vi "Extract Capacity Rows.vi"(10 "Row":i32, 11 "all rows":string[][](array[string])) -> (3 "Capacity Data":T1)   [LabVIEW 2012]
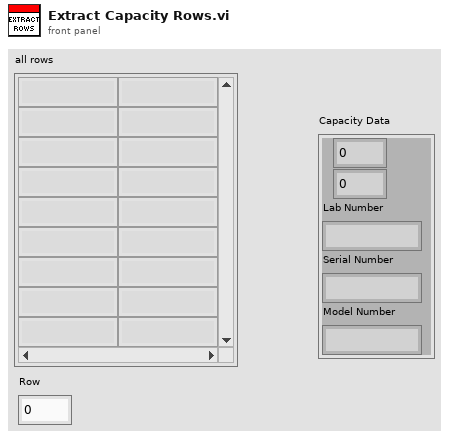
[diagram p1: front panel]
types:
  T1 = cluster{"Measured Temp":dbl, "Weight of Water":dbl, "Lab Number":string, "Serial Number":string, "Model Number":string}
  T2 = cluster{dbl, dbl, "String":string, "String":string, "String":string}
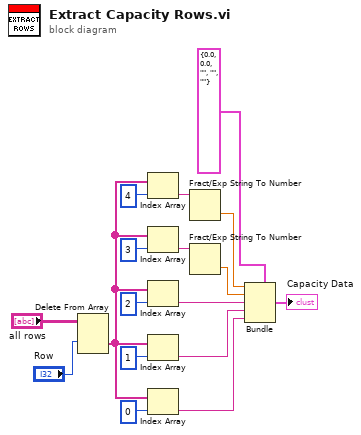
[diagram p0: block diagram]
diagram:
  n1 = Delete From Array(array="all rows", index (row)="Row") -> (deleted portion=w9:string[])  [unwired: 2 in, 1 out]
  n2 = Index Array(array=w9, index=4) -> (element=w16:string)
  n3 = Index Array(array=w9, index=3) -> (element=w15:string)
  n4 = Index Array(array=w9, index=2) -> (element=w5:string)
  n5 = Index Array(array=w9, index=1) -> (element=w4:string)
  n6 = Index Array(array=w9, index=0) -> (element=w3:string)
  n7 = Fract/Exp String To Number(string=w16) -> (number=w7:dbl)  [unwired: 3 in, 1 out]
  n8 = Fract/Exp String To Number(string=w15) -> (number=w6:dbl)  [unwired: 3 in, 1 out]
  n9 = Bundle(cluster=T2 {0.0, 0.0, "String"="", "String"="", "String"=""}, w7, w6, "String"=w5, "String"=w4, "String"=w3) -> (→"Capacity Data":T2)
